vi "convert_path.vi"(8 "error in (no error)":errorcluster, 9 "key array in":string[](array[string]), 10 "xpath in":string) -> (0 "error out":errorcluster, 1 "xpath out":string, 2 "key array out":string[](array[string]))   [LabVIEW 2011, in "XMLElement.lvclass"]
uses:
  XMLElement.lvclass
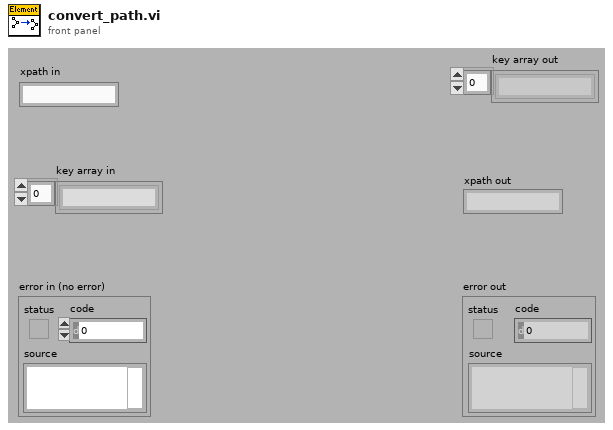
[diagram p1: front panel]
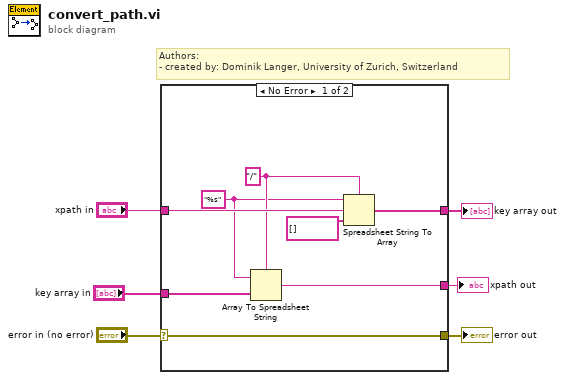
[diagram p0: block diagram]
diagram:
  # "Authors: \n- created by: Dominik Langer, University of Zurich, Switzerland"
  n1 = case shown="No Error" "error in (no error)" {
    selector: "error in (no error)" -> [w14 w15]
    tunnel: [w14 w15] -> w5
    tunnel: "xpath in" -> [w13 _]
    tunnel: [w11 _] -> w3
    tunnel: "key array in" -> [w10 _]
    tunnel: [w7 _] -> w1
    frame No Error {
      w9 = "/" ("delimiter (Tab)")
      w8 = "%s" ("format string")
      n2 = Array To Spreadsheet String(delimiter (Tab)=w9, array=w10, 3:w8) -> (spreadsheet string=w7:string)
      n3 = Spreadsheet String To Array(delimiter (Tab)=w9, format string=w8, spreadsheet string=w13, array type (2D Dbl)=string[] []) -> (array=w11:string[])
    }
    frame Error {
    }
  }
  "error out" <- w5
  "key array out" <- w3
  "xpath out" <- w1
